vi "Read Analog.vi"(8 "error in (no error)":errorcluster, 10 "Params":variant, 11 "NI Analog Input in":refnum<class "NI Analog Input.lvclass">) -> (0 "error out":errorcluster, 2 "Data":variant, 3 "NI Analog Input out":refnum<class "NI Analog Input.lvclass">)   [LabVIEW 2020, in "NI DAQmx.lvlib" / "NI Analog Input.lvclass"]
uses:
  NI Analog Input.lvclass
  D:/WSGitHub/RTFWK/Realization/NI DAQmx Base/NI DAQmx Base.lvclass
  <vilib>/DAQmx/read.llb/DAQmx Read (Analog 1D DBL 1Chan NSamp).vi
  <vilib>/DAQmx/read.llb/DAQmx Read (Analog DBL 1Chan 1Samp).vi
  <vilib>/DAQmx/read.llb/DAQmx Read (Analog 2D DBL NChan NSamp).vi
  <vilib>/DAQmx/read.llb/DAQmx Read (Analog 1D DBL NChan 1Samp).vi
  <vilib>/DAQmx/miscellaneous.llb/DAQmx Fill In Error Info.vi
  <resource>/objmgr/daqmx.rc
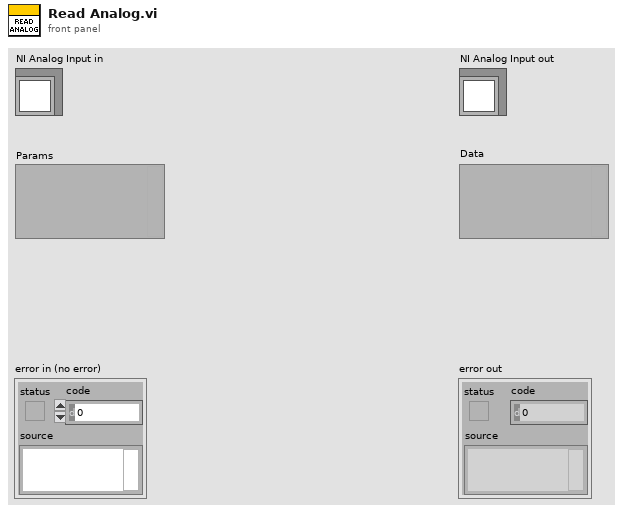
[diagram p1: front panel]
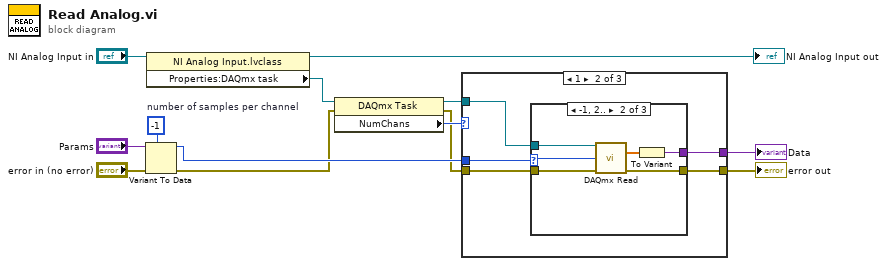
[diagram p0: block diagram]
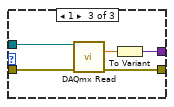
[diagram p4: hidden frame]
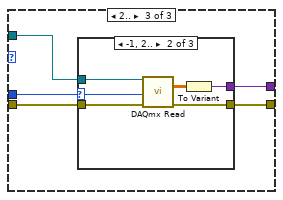
[diagram p5: hidden frame]
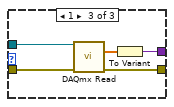
[diagram p7: hidden frame]
diagram:
  w7 = -1  # number of samples per channel
  n1 = Variant To Data(error in="error in (no error)", type=w7, Variant="Params") -> (data=w3:i32, error out=w2:errorcluster)
  n2 = property class="NI Analog Input.lvclass"(reference="NI Analog Input in") -> (reference out=→"NI Analog Input out":refnum<class "NI Analog Input.lvclass">, "Properties:DAQmx task"=w8:refnum<k21>)  [unwired: 1 in, 1 out]
  n3 = property class="DAQmx Task"(reference=w8, error in=w2) -> (reference out=w9:refnum<k21>, error out=w1:errorcluster, "NumChans"=w11:u32)
  n4 = case shown="1" w11 {
    tunnel: [w14 w18 w35] -> w10
    tunnel: w1 -> [w14 w19 w36]
    tunnel: w9 -> [_ w17 w34]
    tunnel: [_ w16 w33] -> w5
    tunnel: w3 -> [_ w15 w32]
    frame 0, Default {
    }
    frame 1 {
      n5 = case shown="-1, 2.." w15 {
        selector: w15 -> [_ w21 _]
        tunnel: w19 -> [w20 w26 w31]
        tunnel: [w20 w25 w30] -> w18
        tunnel: w17 -> [_ w24 w29]
        tunnel: [_ w22 w27] -> w16
        frame 0, Default {
        }
        frame -1, 2.. {
          n6 = call-poly <vilib>:"DAQmx Read.vi"("task/channels in"=w24, "number of samples per channel"=w21, "error in"=w26) -> ("data"=w23:dbl[], "error out"=w25:errorcluster)  [unwired: 10 in, 1 out]
          n7 = To Variant(anything=w23) -> (Variant=w22:variant)
        }
        frame 1 {
          n8 = call-poly <vilib>:"DAQmx Read.vi"("task/channels in"=w29, "error in"=w31) -> ("data"=w28:dbl, "error out"=w30:errorcluster)  [unwired: 11 in, 1 out]
          n9 = To Variant(anything=w28) -> (Variant=w27:variant)
        }
      }
    }
    frame 2.. {
      n10 = case shown="-1, 2.." w32 {
        selector: w32 -> [_ w38 _]
        tunnel: w36 -> [w37 w43 w48]
        tunnel: [w37 w42 w47] -> w35
        tunnel: w34 -> [_ w41 w46]
        tunnel: [_ w39 w44] -> w33
        frame 0, Default {
        }
        frame -1, 2.. {
          n11 = call-poly <vilib>:"DAQmx Read.vi"("task/channels in"=w41, "number of samples per channel"=w38, "error in"=w43) -> ("data"=w40:dbl[][], "error out"=w42:errorcluster)  [unwired: 10 in, 1 out]
          n12 = To Variant(anything=w40) -> (Variant=w39:variant)
        }
        frame 1 {
          n13 = call-poly <vilib>:"DAQmx Read.vi"("task/channels in"=w46, "error in"=w48) -> ("data"=w45:dbl[], "error out"=w47:errorcluster)  [unwired: 11 in, 1 out]
          n14 = To Variant(anything=w45) -> (Variant=w44:variant)
        }
      }
    }
  }
  "error out" <- w10
  "Data" <- w5
